vi "arcus main.vi"(0 "Communication Port":refnum<visa-resource-name>="COM5", 1 "Device Address":string="*IDN?\r\n", 2 "Command":string) -> (10 "Response":string)   [LabVIEW 2013]
doc: "The Basic Serial Read and Write example performs a Serial Port Read, a Serial Port Write, or a combination of these actions. The user selects the actions (read or write) on the front panel. If both are selected, the VI will write the data first, read data, and then close the VISA session that is opened to the port. This VI will wait until the specified number of bytes is received at the port. Only the number of bytes specified will be read.\n\nINSTRUCTIONS:\n1) Select the serial resource and configuration parameters (baud rate, data bits, parity, stop bits, flow control).\n2) Select the operations to be performed. \n3) Connect the serial port to your device. If no device is available, perform a loopback test by doing one of the following. Short pins 2 and 3 on a RS-232 cable or short pin 4 to pin 8 and pin 5 to pin 9 on a RS-485/422 cable. \n4) Run the VI to see the data read. (The \"read string\" will match the \"string to write\" if a loopback test was performed.)\n\nNote: The parameters set for the serial port must match the parameters of the connected instrument or device. In this example, the bytes to read parameter specifies the number of bytes that the serial port reads. If there were more bytes at the port than the number specified in bytes to read, those bytes would not be read. Also, if you specify to read more bytes than the number of bytes actually read, you might receive a timeout error message.\n\nOn the block diagram, the Configure Serial Port VI sets the configuration parameters. The front panel displays the controls used to configure the basic parameters, such as baud rate, data bits, and parity. Constants configure the other parameters the user probably does not need set. After the VISA Configure Serial Port VI opens the VISA session and configures the port, the VI passes the VISA resource name to other VIs that perform operations on that VISA resource. The VISA Write function sends a command to the serial device and the VISA Read function returns data based on the command. The VISA Close function then closes the reference to the serial device. It is important to close the reference; otherwise communication through with that port through protocols other than VISA might not be possible."
uses:
  <vilib>/Instr/_visa.llb/VISA Configure Serial Port (Instr).vi
panel:
  in  "Baud Rate":u32=9600
  # "Communication Setup"
  # "Send/Receive Commands"
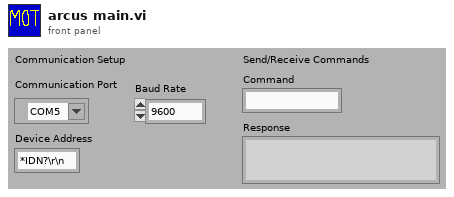
[diagram p1: front panel]
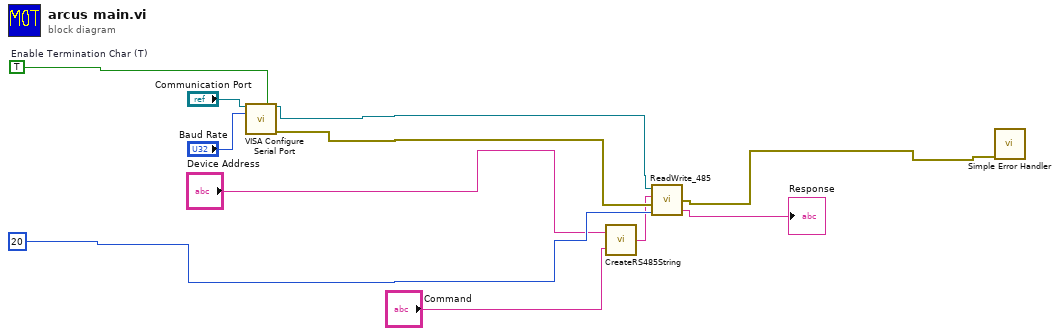
[diagram p0: block diagram]
diagram:
  w10 = TRUE  # Enable Termination Char (T)
  n1 = call-poly "VISA Configure Serial Port"("VISA resource name"="Communication Port", "Enable Termination\nChar (T)"=w10, "baud rate (9600)"="Baud Rate") -> ("VISA resource name out"=w8:refnum<visa-resource-name>, "error out"=w7:errorcluster)  [unwired: 11 in]
  n2 = call "CreateRS485String.vi"("Command"="Command", "Address"="Device Address") -> ("Output String"=w2:string)
  n3 = call "ReadWrite_485.vi"("delay before read (ms)"=20, "error in"=w7, "Command"=w2, "VISA In"=w8) -> ("Response"=→"Response":string, "error out"=w9:errorcluster)  [unwired: 1 out]
  n4 = call <vilib>:"Simple Error Handler.vi"("error in (no error)"=w9) -> ()  [unwired: 4 in, 5 out]
